vi "2DSimulator_Inverse_Kinematics.vi"() -> ()   [LabVIEW 2024]
panel:
  in  "?":bool
  in  "Delay":dbl(slide) scale=100.0..1000.0
  out "Bot Arm":picture
  in  "Colors":T1={"Base"=16750848, "Link 1"=16764006, "Joint 2"=26316, "Link 2"=6723993, "EOF"=16724787}
  out "Length 1":dbl
  out "Length 2":dbl
  out "Angle 2":dbl
  out "Angle 1":dbl
  # "L2"
  # "Overview: This VI demonstrates the inverse kinematics function for a 2DOF Bot used in ME121 Advanced Dynamics for the spring semester 2025, Tufts University. This VI draws a crab using the end-of-effector\n\nInstructions: \n1. Run the VI.\n2. The user will be able to visualize the motion of the arm to draw a crab and the parameters associated to the angles and lengths of each link. The user can also speed up or slow down the motion. \n3. Click Stop to stop the VI."
  # "Angle 2"
  # "Angle 1"
  # "L1"
  # "Crab Shape"
  # "Lengths of links (mm)"
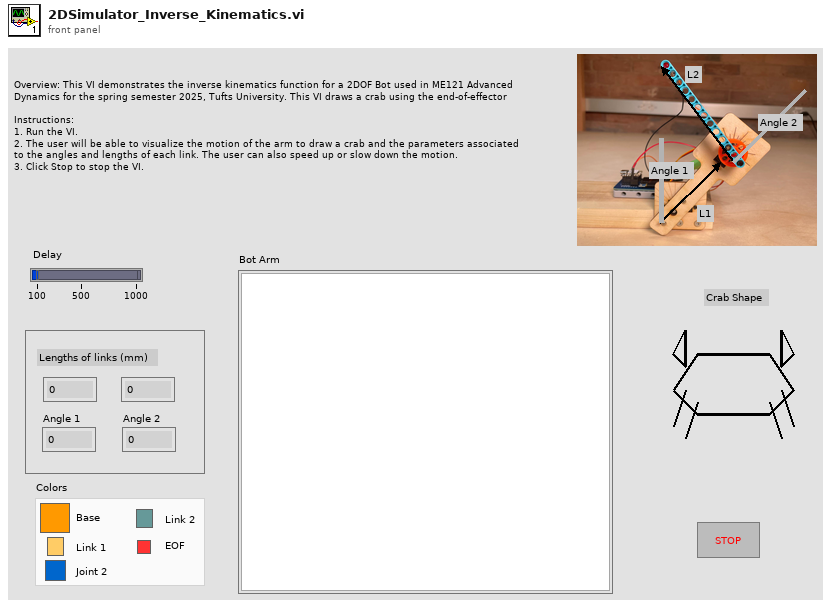
[diagram p1: front panel]
types:
  T1 = cluster{"Base":u32, "Link 1":u32, "Joint 2":u32, "Link 2":u32, "EOF":u32}
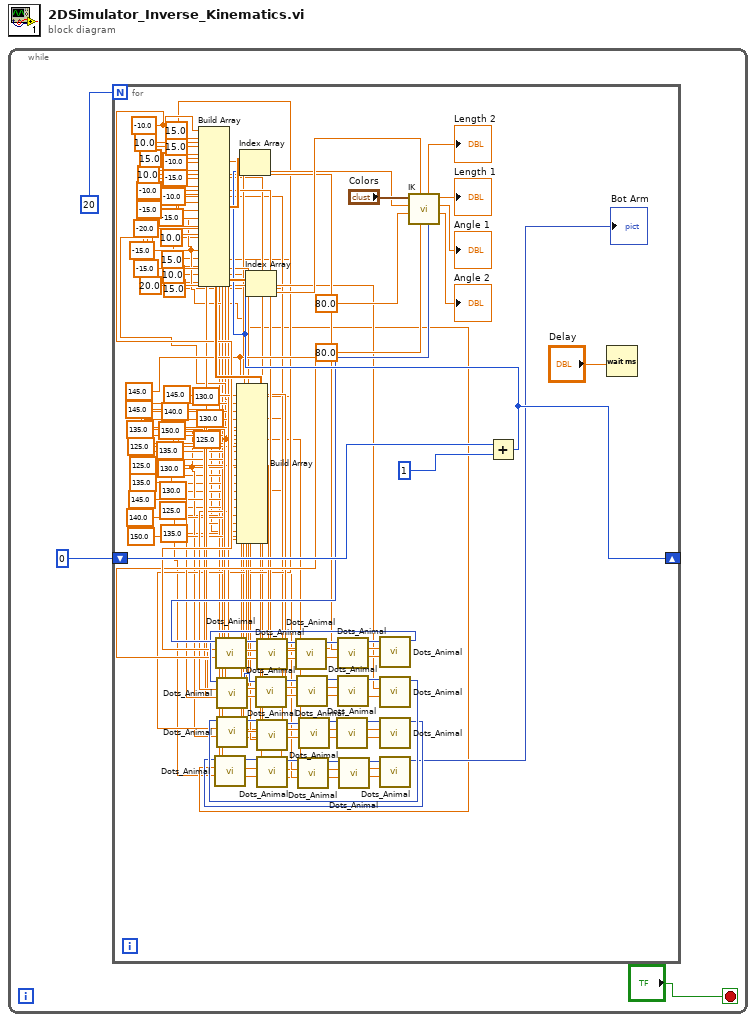
[diagram p0: block diagram]
diagram:
  n1 = while {
    stop <- "?" stop-if-true
    n2 = for {
      N: 20 -> [_]
      shift-right: [w68] -> _
      shift-left: 0 -> [w72]
      w4 = 125.0 ("element")
      w5 = 15.0 ("element")
      w7 = 10.0 ("element")
      w9 = 15.0 ("element")
      w11 = 10.0 ("element")
      w13 = -15.0 ("element")
      w15 = -10.0 ("element")
      w17 = -15.0 ("element")
      w19 = -10.0 ("element")
      w21 = 15.0 ("element")
      w23 = 15.0 ("element")
      w6 = 130.0 ("element")
      w8 = 130.0 ("element")
      w10 = 135.0 ("element")
      w12 = 125.0 ("element")
      w14 = 130.0 ("element")
      w16 = 130.0 ("element")
      w18 = 135.0 ("element")
      w20 = 150.0 ("element")
      w22 = 140.0 ("element")
      w24 = 145.0 ("element")
      w25 = 20.0 ("element")
      w27 = -15.0 ("element")
      w29 = -15.0 ("element")
      w31 = -20.0 ("element")
      w33 = -15.0 ("element")
      w35 = -10.0 ("element")
      w37 = 10.0 ("element")
      w39 = 15.0 ("element")
      w41 = 10.0 ("element")
      w26 = 150.0 ("element")
      w28 = 140.0 ("element")
      w30 = 145.0 ("element")
      w32 = 135.0 ("element")
      w34 = 125.0 ("element")
      w36 = 125.0 ("element")
      w38 = 135.0 ("element")
      w40 = 145.0 ("element")
      w43 = -10.0 ("element")
      w42 = 145.0 ("element")
      n3 = Build Array(w43, w41, w39, w37, w35, w33, w31, w29, w27, w25, w23, w21, w19, w17, w15, w13, w11, w9, w7, w5) -> (w69:dbl[])
      n4 = Build Array(w42, w40, w38, w36, w34, w32, w30, w28, w26, w24, w22, w20, w18, w16, w14, w12, w10, w8, w6, w4) -> (w70:dbl[])
      n5 = Add(x=w72, y=1) -> (x+y=w68:i32)
      n6 = Index Array(array=w69, index=w68) -> (element=w66:dbl)
      n7 = Index Array(array=w70, index=w68) -> (element=w67:dbl)
      n8 = call "IK.vi"("Length 4"=80.0 ("Length 2"), "Y Coordinate"=w67, "Length 3"=80.0 ("Length 1"), "X Coordinate"=w66, "Colors"="Colors") -> ("Angle 2"=→"Angle 2":dbl, "Angle 1"=→"Angle 1":dbl, "Length 1"=→"Length 1":dbl, "Picture Out"=w64:picture, "Length 2"=→"Length 2":dbl)  [unwired: 2 in]
      n9 = call "Dots_Animal.vi"("element"=w42, "element 2"=w43, "Picture Out"=w64) -> ("new picture"=w63:picture)  [unwired: 8 in]
      n10 = call "Dots_Animal.vi"("element"=w40, "element 2"=w41, "Picture Out"=w63) -> ("new picture"=w62:picture)  [unwired: 8 in]
      n11 = call "Dots_Animal.vi"("element"=w38, "element 2"=w39, "Picture Out"=w62) -> ("new picture"=w61:picture)  [unwired: 8 in]
      n12 = call "Dots_Animal.vi"("element"=w36, "element 2"=w37, "Picture Out"=w61) -> ("new picture"=w60:picture)  [unwired: 8 in]
      n13 = call "Dots_Animal.vi"("element"=w34, "element 2"=w35, "Picture Out"=w60) -> ("new picture"=w59:picture)  [unwired: 8 in]
      n14 = call "Dots_Animal.vi"("element"=w32, "element 2"=w33, "Picture Out"=w59) -> ("new picture"=w58:picture)  [unwired: 8 in]
      n15 = call "Dots_Animal.vi"("element"=w30, "element 2"=w31, "Picture Out"=w58) -> ("new picture"=w57:picture)  [unwired: 8 in]
      n16 = call "Dots_Animal.vi"("element"=w28, "element 2"=w29, "Picture Out"=w57) -> ("new picture"=w56:picture)  [unwired: 8 in]
      n17 = call "Dots_Animal.vi"("element"=w26, "element 2"=w27, "Picture Out"=w56) -> ("new picture"=w55:picture)  [unwired: 8 in]
      n18 = call "Dots_Animal.vi"("element"=w24, "element 2"=w25, "Picture Out"=w55) -> ("new picture"=w54:picture)  [unwired: 8 in]
      n19 = call "Dots_Animal.vi"("element"=w22, "element 2"=w23, "Picture Out"=w54) -> ("new picture"=w53:picture)  [unwired: 8 in]
      n20 = call "Dots_Animal.vi"("element"=w20, "element 2"=w21, "Picture Out"=w53) -> ("new picture"=w52:picture)  [unwired: 8 in]
      n21 = call "Dots_Animal.vi"("element"=w18, "element 2"=w19, "Picture Out"=w52) -> ("new picture"=w51:picture)  [unwired: 8 in]
      n22 = call "Dots_Animal.vi"("element"=w16, "element 2"=w17, "Picture Out"=w51) -> ("new picture"=w50:picture)  [unwired: 8 in]
      n23 = call "Dots_Animal.vi"("element"=w14, "element 2"=w15, "Picture Out"=w50) -> ("new picture"=w49:picture)  [unwired: 8 in]
      n24 = call "Dots_Animal.vi"("element"=w12, "element 2"=w13, "Picture Out"=w49) -> ("new picture"=w48:picture)  [unwired: 8 in]
      n25 = call "Dots_Animal.vi"("element"=w10, "element 2"=w11, "Picture Out"=w48) -> ("new picture"=w47:picture)  [unwired: 8 in]
      n26 = call "Dots_Animal.vi"("element"=w8, "element 2"=w9, "Picture Out"=w47) -> ("new picture"=w46:picture)  [unwired: 8 in]
      n27 = call "Dots_Animal.vi"("element"=w6, "element 2"=w7, "Picture Out"=w46) -> ("new picture"=w45:picture)  [unwired: 8 in]
      n28 = call "Dots_Animal.vi"("element"=w4, "element 2"=w5, "Picture Out"=w45) -> ("new picture"=→"Bot Arm":picture)  [unwired: 8 in]
      n29 = Wait (ms)(milliseconds to wait="Delay") -> ()  [unwired: 1 out]
    }
  }
